vi "Get ImageData.vi"(8 "error in (no error)":errorcluster, 10 "GetElement (-1: Current)":i32=-1, 11 "CircularBuffer.ImageData":refnum<class "CircularBuffer.ImageData.lvclass">) -> (0 "error out":errorcluster, 2 "ImageData":T1, 3 "CircularBuffer.ImageData out":refnum<class "CircularBuffer.ImageData.lvclass">)   [LabVIEW 2015, in "CircularBuffer.ImageData.lvclass"]
uses:
  CircularBuffer.ImageData.lvclass
  <vilib>/picture/picture.llb/imagedata.ctl
  CircularBuffer/CircularBuffer.lvclass
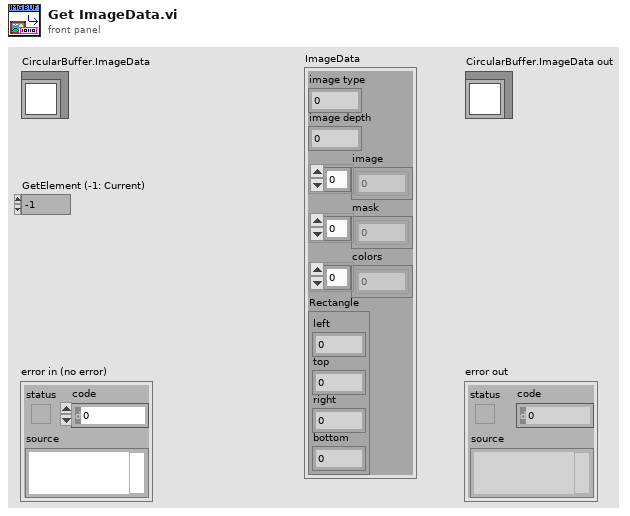
[diagram p1: front panel]
types:
  T1 = typedef "imagedata.ctl" = cluster{"image type":i32, "image depth":i32, "image":u8[], "mask":u8[], "colors":u32[], "Rectangle":cluster{"left":i16, "top":i16, "right":i16, "bottom":i16}}
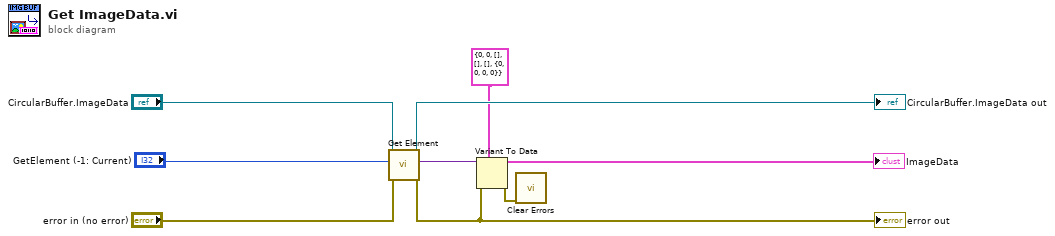
[diagram p0: block diagram]
diagram:
  n1 = call "Get Element.vi"("error in (no error)"="error in (no error)", "GetElement (-1: Current)"="GetElement (-1: Current)", "CircularBuffer"="CircularBuffer.ImageData") -> ("error out"=w1:errorcluster, "Element"=w7:variant, "CircularBuffer out"=→"CircularBuffer.ImageData out":refnum<class "CircularBuffer.ImageData.lvclass">)  [unwired: 6 in]
  "error out" <- w1
  n2 = Variant To Data(error in=w1, type=T1 {"image type"=0, "image depth"=0, "image"=[], "mask"=[], "colors"=[], "Rectangle"={"left"=0, "top"=0, "right"=0, "bottom"=0}} ("ImageData"), Variant=w7) -> (data=→"ImageData":T1, error out=w3:errorcluster)
  n3 = call <vilib>:"Clear Errors.vi"("error in (no error)"=w3) -> ()  [unwired: 5 in, 2 out]
